vi "PH_PILS.PC _Status Emergency off changed.vi"(0 "i ref in":refnum<vi>, 5 "error in":errorcluster) -> (14 "i ref out":refnum<vi>, 19 "error out":errorcluster)   [LabVIEW 2014, in "PH_PILS.lvlib"]
uses:
  PH_PILS.lvlib
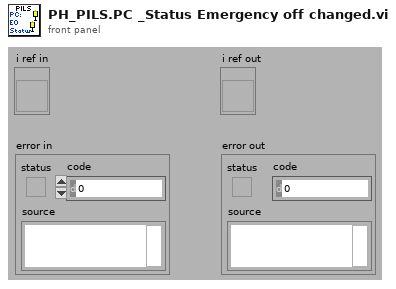
[diagram p1: front panel]
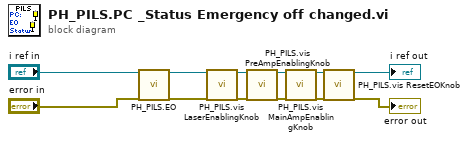
[diagram p0: block diagram]
diagram:
  n1 = call "PH_PILS.EO.vi"("i ref in"="i ref in", "error in"="error in") -> ("i ref out"=w1:refnum<vi>, "error out"=w3:errorcluster)  [unwired: 16 in]
  n2 = call "PH_PILS.vis LaserEnablingKnob.vi"("i ref in"=w1, "error IO"=w3) -> ("i ref out"=w11:refnum<vi>, "error out"=w12:errorcluster)  [unwired: 16 in]
  n3 = call "PH_PILS.vis PreAmpEnablingKnob.vi"("i ref in"=w11, "error IO"=w12) -> ("i ref out"=w9:refnum<vi>, "error out"=w10:errorcluster)  [unwired: 16 in]
  n4 = call "PH_PILS.vis MainAmpEnablingKnob.vi"("i ref in"=w9, "error IO"=w10) -> ("i ref out"=w8:refnum<vi>, "error out"=w7:errorcluster)  [unwired: 16 in]
  n5 = call "PH_PILS.vis ResetEOKnob.vi"("i ref in"=w8, "error IO"=w7) -> ("i ref out"=→"i ref out":refnum<vi>, "error out"=→"error out":errorcluster)  [unwired: 16 in]
